vi "Build Menu.vi"(8 "error in (no error)":errorcluster, 11 "menu reference":refnum<k9>) -> (0 "error out":errorcluster, 2 "Station Config":T1, 3 "element":string)   [LabVIEW 2025, in "Full User Interface.lvlib"]
uses:
  Full User Interface.lvlib
  Station Config.ctl
  Station Info.ctl
  <vilib>/Utility/miscctls.llb/LVMenuShortCut.ctl
  Key.ctl
  Localization/Section.ctl
  Localization/Localization.lvlib
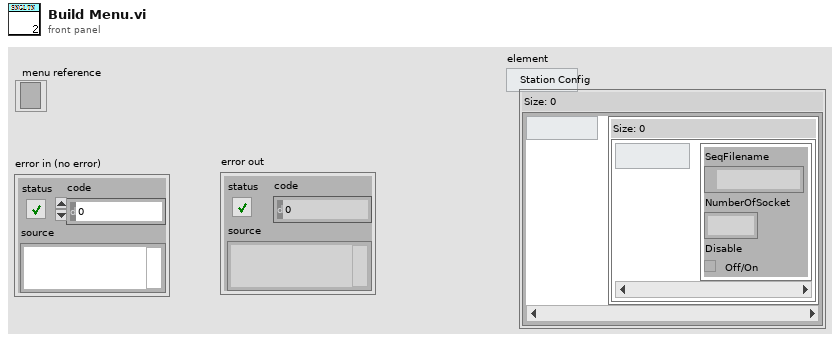
[diagram p1: front panel]
types:
  T1 = typedef "Full User Interface.lvlib/Station Config.ctl" = map{string, map{i32, T2}}
  T2 = typedef "Full User Interface.lvlib/Station Info.ctl" = cluster{"SeqFilename":path, "NumberOfSocket":i32, "Disable":bool}
  T3 = typedef "Localization.lvlib/Section.ctl" = enum16{"Menu", "Title", "Workstation Config"}
  T4 = typedef "Full User Interface.lvlib/Key.ctl" = enum16{"Language", "Model"}
  T5 = typedef "LVMenuShortCut.ctl" = cluster{"Include Shift Key?":bool, "Include Ctrl Key?":bool, "Shortcut Key":string}
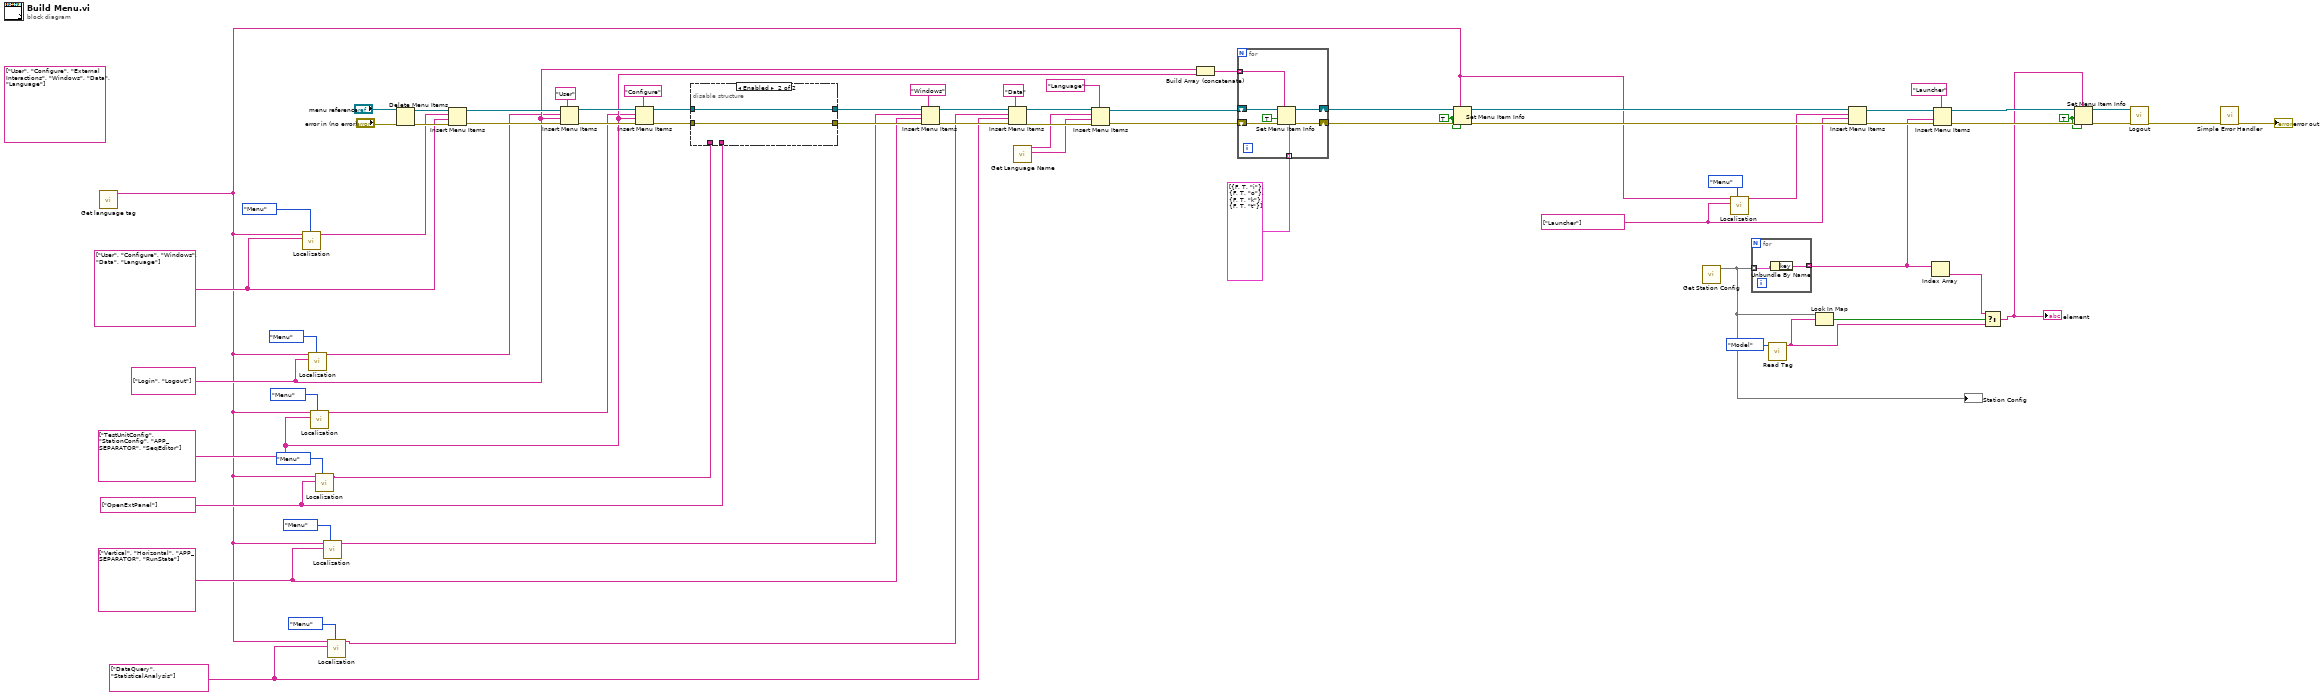
[diagram p0: block diagram]
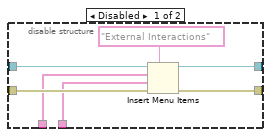
[diagram p2: hidden frame]
diagram:
  (unwired) string[] ["User", "Configure", "External Interactions", "Windows", "Data", "Language"] ("item tags")
  w17 = TRUE ("enabled")
  w30 = TRUE ("enabled")
  w3 = string[] ["DataQuery", "StatisticalAnalysis"]
  w7 = string[] ["Vertical", "Horizontal", "APP_SEPARATOR", "RunState"]
  w10 = string[] ["OpenExtPanel"]
  w26 = string[] ["Launcher"]
  w29 = string[] ["User", "Configure", "Windows", "Data", "Language"] ("item tags")
  w13 = string[] ["TestUnitConfig", "StationConfig", "APP_SEPARATOR", "SeqEditor"] ("item tags")
  w16 = string[] ["Login", "Logout"] ("item tags")
  n1 = call "Get language tag.vi"() -> ("language tag"=w4:string)  [unwired: 11 in]
  n2 = call "Localization.vi"("section"=Section."Menu", "key"=w29, "Language key"=w4) -> ("Value"=w28:string[])  [unwired: 7 in, 1 out]
  n3 = call "Localization.vi"("section"=Section."Menu", "key"=w16, "Language key"=w4) -> ("Value"=w15:string[])  [unwired: 7 in, 1 out]
  n4 = call "Localization.vi"("section"=Section."Menu", "key"=w13, "Language key"=w4) -> ("Value"=w12:string[])  [unwired: 7 in, 1 out]
  n5 = call "Localization.vi"("section"=Section."Menu", "key"=w10, "Language key"=w4) -> ("Value"=w8:string[])  [unwired: 7 in, 1 out]
  n6 = call "Localization.vi"("section"=Section."Menu", "key"=w7, "Language key"=w4) -> ("Value"=w5:string[])  [unwired: 7 in, 1 out]
  n7 = call "Localization.vi"("section"=Section."Menu", "key"=w3, "Language key"=w4) -> ("Value"=w1:string[])  [unwired: 7 in, 1 out]
  n8 = Delete Menu Items(6:"error in (no error)", 9:"menu reference") -> (0:w61:errorcluster, 3:w60:refnum<k9>)  [unwired: 2 in]
  n9 = Insert Menu Items(6:w61, 7:w29, 8:w28, 9:w60) -> (0:w65:errorcluster, 3:w66:refnum<k9>)  [unwired: 2 in, 1 out]
  n10 = Insert Menu Items(5:"User" ("menu tag"), 6:w65, 7:w16, 8:w15, 9:w66) -> (0:w69:errorcluster, 3:w70:refnum<k9>)  [unwired: 1 in, 1 out]
  n11 = Insert Menu Items(5:"Configure" ("menu tag"), 6:w69, 7:w13, 8:w12, 9:w70) -> (0:w52:errorcluster, 3:w53:refnum<k9>)  [unwired: 1 in, 1 out]
  n12 = disable-structure shown="Enabled" {
    disable-tunnel: w53 -> [w78 w80]
    disable-tunnel: w52 -> [w77 w79]
    disable-tunnel: [w75 w80] -> w51
    disable-tunnel: [w74 w79] -> w50
    disable-tunnel: w10 -> [w73 _]
    disable-tunnel: w8 -> [w72 _]
    frame Disabled {
      n13 = Insert Menu Items(5:"External Interactions", 6:w77, 7:w73, 8:w72, 9:w78) -> (0:w74:errorcluster, 3:w75:refnum<k9>)  [unwired: 1 in, 1 out]
    }
    frame Enabled {
    }
  }
  n14 = Insert Menu Items(5:"Windows", 6:w50, 7:w7, 8:w5, 9:w51) -> (0:w43:errorcluster, 3:w44:refnum<k9>)  [unwired: 1 in, 1 out]
  n15 = Insert Menu Items(5:"Data", 6:w43, 7:w3, 8:w1, 9:w44) -> (0:w38:errorcluster, 3:w41:refnum<k9>)  [unwired: 1 in, 1 out]
  n16 = call "Get Language Name.vi"() -> ("Tag"=w31:string[], "Tag Name"=w32:string[])  [unwired: 8 in, 2 out]
  n17 = Insert Menu Items(5:"Language", 6:w38, 7:w31, 8:w32, 9:w41) -> (0:w39:errorcluster, 3:w40:refnum<k9>)  [unwired: 1 in, 1 out]
  n18 = Build Array (concatenate)(w16, w13) -> (w67:string[])
  n19 = for {
    shift-right: [w86] -> w36
    shift-left: w40 -> [w87]
    shift-right: [w84] -> w35
    shift-left: w39 -> [w85]
    tunnel: w67 -> [w83] mode=indexing
    tunnel: T5[] [{"Include Shift Key?"=FALSE, "Include Ctrl Key?"=TRUE, "Shortcut Key"="i"}, {"Include Shift Key?"=FALSE, "Include Ctrl Key?"=TRUE, "Shortcut Key"="o"}, {"Include Shift Key?"=FALSE, "Include Ctrl Key?"=TRUE, "Shortcut Key"="k"}, {"Include Shift Key?"=FALSE, "Include Ctrl Key?"=TRUE, "Shortcut Key"="t"}] -> [w81] mode=indexing
    n20 = Set Menu Item Info(4:w81, 7:w83, 8:w85, 9:TRUE ("enabled"), 11:w87) -> (0:w84:errorcluster, 3:w86:refnum<k9>)  [unwired: 2 in]
  }
  n21 = Set Menu Item Info(6:w30, 7:w4, 8:w35, 9:w30, 11:w36) -> (0:w34:errorcluster, 3:w33:refnum<k9>)  [unwired: 2 in]
  n22 = call "Get Station Config.vi"() -> ("Station Config"=w22:T1)  [unwired: 10 in, 1 out]
  "Station Config" <- w22
  n23 = call "Localization.vi"("section"=Section."Menu", "key"=w26, "Language key"=w4) -> ("Value"=w25:string[])  [unwired: 7 in, 1 out]
  n24 = for {
    tunnel: w22 -> [w89] mode=indexing
    tunnel: [w88] -> w54 mode=indexing
    n25 = Unbundle By Name(w89) -> ("key"=w88:string)
  }
  n26 = call "Read Tag.vi"("Enum"=Key."Model") -> ("value"=w19:string)  [unwired: 9 in, 1 out]
  n27 = Look In Map(map=w22, key=w19) -> (key not found?=w21:bool)  [unwired: 1 in, 1 out]
  n28 = Insert Menu Items(6:w34, 7:w26, 8:w25, 9:w33) -> (0:w59:errorcluster, 3:w57:refnum<k9>)  [unwired: 2 in, 1 out]
  n29 = Index Array(array=w54) -> (element=w20:string)  [unwired: 1 in]
  n30 = Insert Menu Items(5:"Launcher", 6:w59, 7:w54, 9:w57) -> (0:w56:errorcluster, 3:w55:refnum<k9>)  [unwired: 2 in, 1 out]
  n31 = Select(t=w20, s=w21, f=w19) -> (s? t:f=w18:string)
  "element" <- w18
  n32 = Set Menu Item Info(6:w17, 7:w18, 8:w56, 9:w17, 11:w55) -> (0:w47:errorcluster, 3:w48:refnum<k9>)  [unwired: 2 in]
  n33 = call "Logout.vi"("Error In"=w47, "menu reference"=w48) -> ("Error Out"=w46:errorcluster)  [unwired: 9 in]
  n34 = call <vilib>:"Simple Error Handler.vi"("error in (no error)"=w46) -> ("error out"=→"error out":errorcluster)  [unwired: 4 in, 4 out]
